vi "FFT_subset.vi"(1 "Hz":dbl, 2 "input":dbl[][](array[numeric])) -> (0 "subarray":dbl[][](array[numeric]))   [LabVIEW 2009]
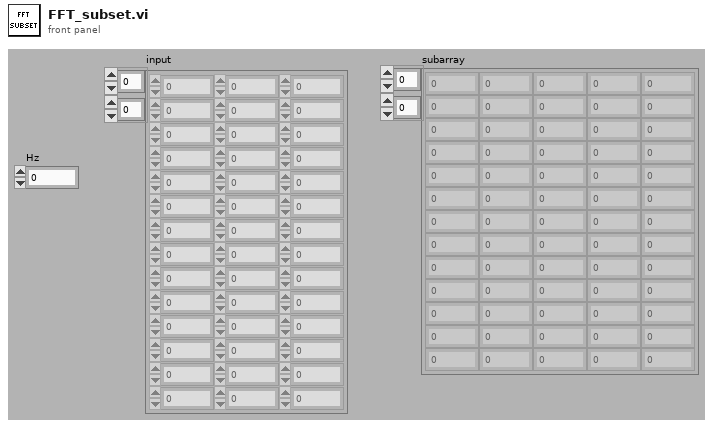
[diagram p1: front panel]
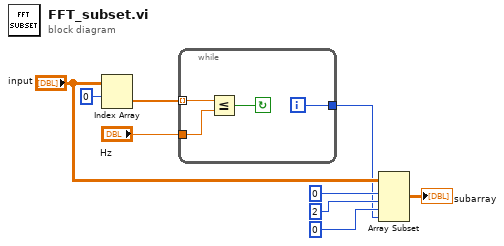
[diagram p0: block diagram]
diagram:
  n1 = Index Array(array="input", index (row)=0) -> (element=w8:dbl[])  [unwired: 1 in]
  n2 = while {
    tunnel: w8 -> [w13] mode=indexing
    tunnel: "Hz" -> [w12]
    tunnel: [w10] -> w2
    i -> [w10]
    stop <- w11 continue-if-true
    n3 = Less Or Equal?(x=w13, y=w12) -> (x <= y?=w11:bool)
  }
  n4 = Array Subset(array="input", index (row)=0 ("index"), length (row)=2 ("length"), index (col)=0 ("index"), length (col)=w2) -> (→"subarray":dbl[][])
